vi "AMDemod.vi"(8 "error in (no error)":errorcluster, 11 "data":waveform(dbl)) -> (0 "error out":errorcluster, 3 "Waveform":waveform(dbl))   [LabVIEW 2018]
uses:
  <vilib>/Analysis/3filter.llb/Filter Passband Type.ctl
  <vilib>/Analysis/3filter.llb/Butterworth Filter (DBL).vi
  <vilib>/Analysis/NI_AALBase.lvlib
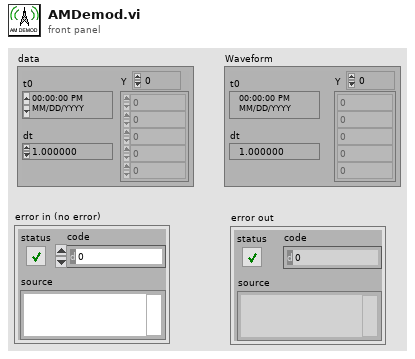
[diagram p1: front panel]
types:
  T1 = typedef "NI_AALBase.lvlib/Filter Passband Type.ctl" = enum32{"Lowpass", "Highpass", "Bandpass", "Bandstop"}
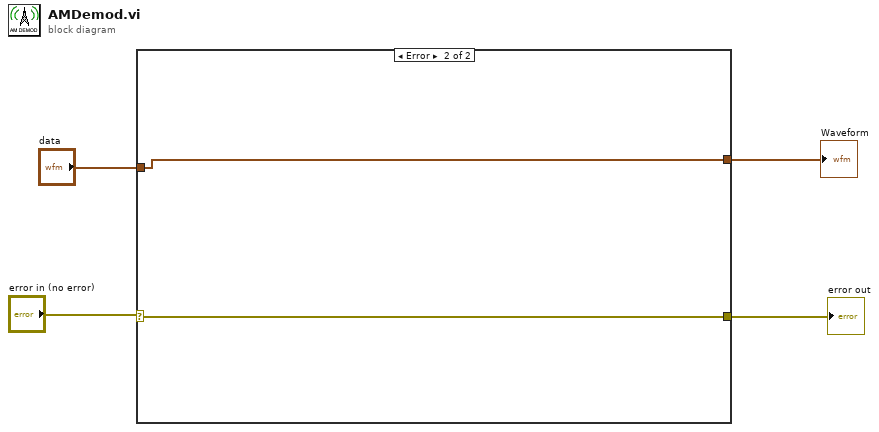
[diagram p0: block diagram]
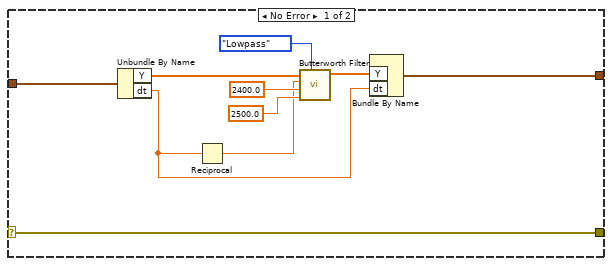
[diagram p2: hidden frame]
diagram:
  n1 = case shown="Error" "error in (no error)" {
    selector: "error in (no error)" -> [w5 w16]
    tunnel: [w14 w15] -> w4
    tunnel: "data" -> [w6 w15]
    tunnel: [w5 w16] -> w1
    frame No Error {
      n2 = Unbundle By Name(w6) -> ("Y"=w7:dbl[], "dt"=w12:dbl)
      n3 = Reciprocal(x=w12) -> (1/x=w9:dbl)
      n4 = call-poly <vilib>:"Butterworth Filter.vi"("filter type"=Filter_Passband_Type."Lowpass", "low cutoff freq: fl"=2500.0, "high cutoff freq: fh"=2400.0, "sampling freq: fs"=w9, "X"=w7) -> ("Filtered X"=w13:dbl[])  [unwired: 3 in, 1 out]
      n5 = Bundle By Name("Y"=w13, "dt"=w12) -> (w14:waveform(dbl))  [unwired: 1 in]
    }
    frame Error {
    }
  }
  "Waveform" <- w4
  "error out" <- w1
